vi "Main.vi"() -> ()   [LabVIEW 2015]
doc: "The boiler controller allows a user to start and shut down a boiler.\n\nUse the Reset, Start, and Light Pilot controls to sequentially start the boiler. \nUse the Fuel Control Valve to change the flow of fuel into the boiler. \nUse the Stop Boiler button to shut down the boiler. \nTo shut down the system or in the event of an emergency, use the Emergency Stop button to close the application completely."
uses:
  controls/MHL Data.ctl
  controls/MHL UI Data.ctl
  controls/MHL Status.ctl
  controls/MHL References.ctl
  controls/MHL Configuration.ctl
  support/Boiler System Globals.vi
  support/Message Queue/Message Queue.lvlib
  support/User Event - Stop/User Event - Stop.lvlib
  Boiler/Boiler.lvlib
panel:
  in  "Fuel Control Valve":u32(slide) scale=10.0..75.0
  in  "Stop Boiler":bool
  in  "Light Pilot":bool
  out "Forced Draft Fan":bool
  out "Pilot":bool
  out "Pilot Gas Valve":bool
  out "Primary Fan":bool
  out "Status":string
  in  "Start":bool
  in  "Reset":bool
  in  "Emergency Stop":bool
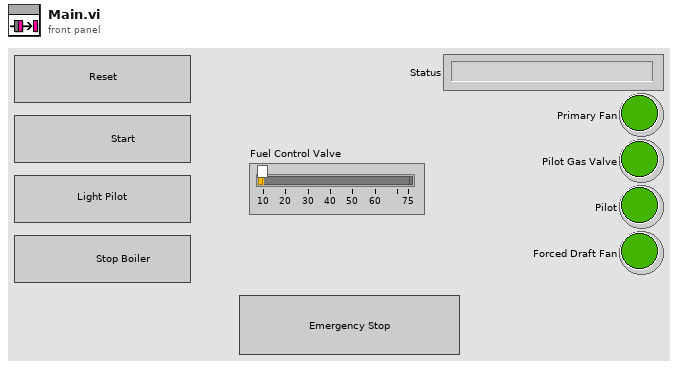
[diagram p1: front panel]
types:
  T1 = typedef "MHL Data.ctl" = cluster{"MHL User Interface Data":T2, "MHL References":T4, "MHL Configuration":T5}
  T2 = typedef "MHL UI Data.ctl" = cluster{"Status":string, "Fuel Control Valve":u32, "Primary Fan":bool, "Pilot Gas Valve":bool, "Pilot":bool, "Forced Draft Fan":bool, "MHL Status":T3}
  T3 = typedef "MHL Status.ctl" = enum16{"Lockout", "Ready", "Pre-Purge", "Pre-Purge Complete", "Pilot On", "Boiler Running", "Shutdown", "Purge"}
  T4 = typedef "MHL References.ctl" = cluster{"Reset Ref":refnum<vi>, "Start Ref":refnum<vi>, "Light Pilot Ref":refnum<vi>, "Stop Boiler Ref":refnum<vi>, "Fuel Control Valve Ref":refnum<vi>}
  T5 = typedef "MHL Configuration.ctl" = cluster{"Fuel Control Valve Maximum":dbl, "Fuel Control Valve Minimum":dbl}
  T6 = typedef "Notifiers.ctl" = cluster{"Handshake":refnum<notifier>, "Flame Level":refnum<notifier>, "Controller Exit":refnum<notifier>, "Boiler Exit":refnum<notifier>}
  T7 = typedef "Message Queue.lvlib/All Message Queues.ctl" = cluster{"MHL":refnum<queue>, "Boiler Controller":refnum<queue>, "Boiler":refnum<queue>}
  T8 = enum32{"invalid app kind", "Development System", "Run Time System", "Student Edition", "Embedded LabVIEW", "Evaluation", "Custom"}
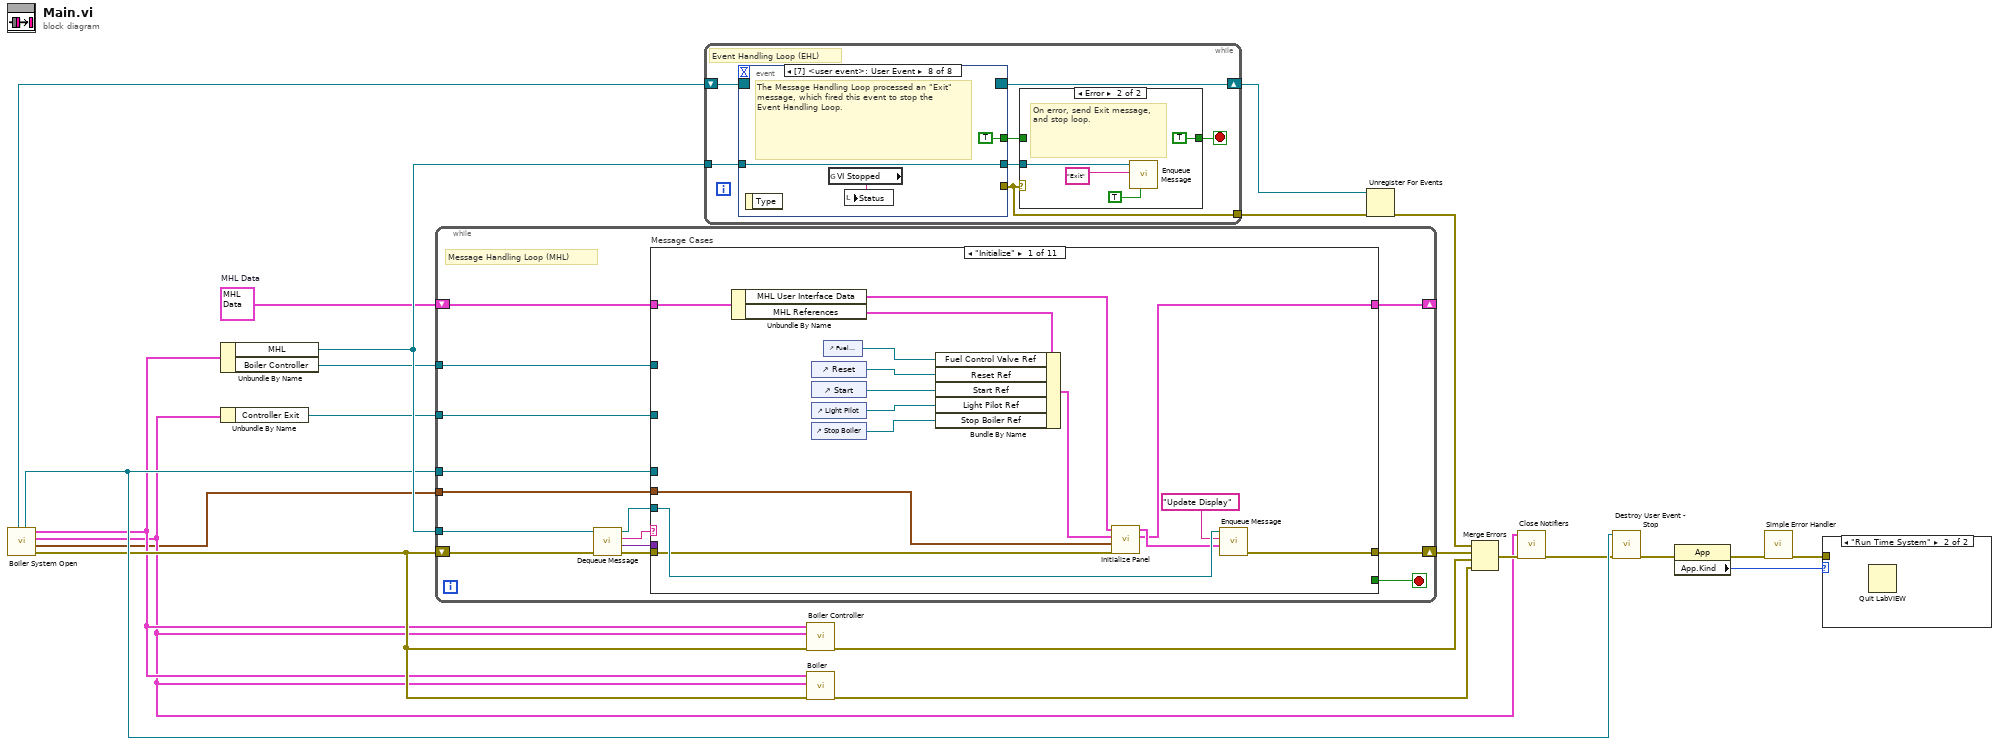
[diagram p0: block diagram]
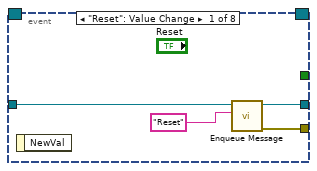
[diagram p4: hidden frame]
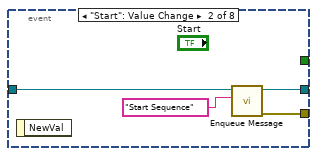
[diagram p5: hidden frame]
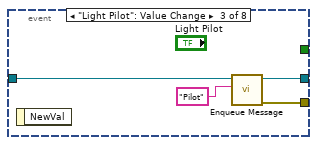
[diagram p6: hidden frame]
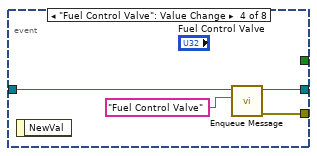
[diagram p7: hidden frame]
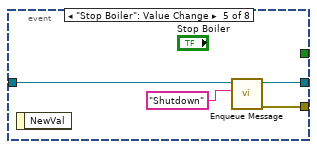
[diagram p8: hidden frame]
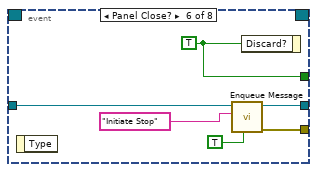
[diagram p9: hidden frame]
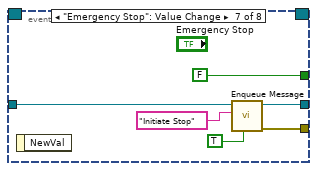
[diagram p10: hidden frame]
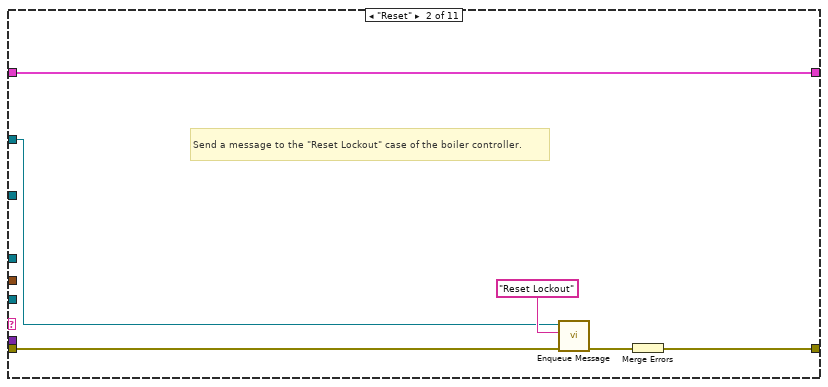
[diagram p11: hidden frame]
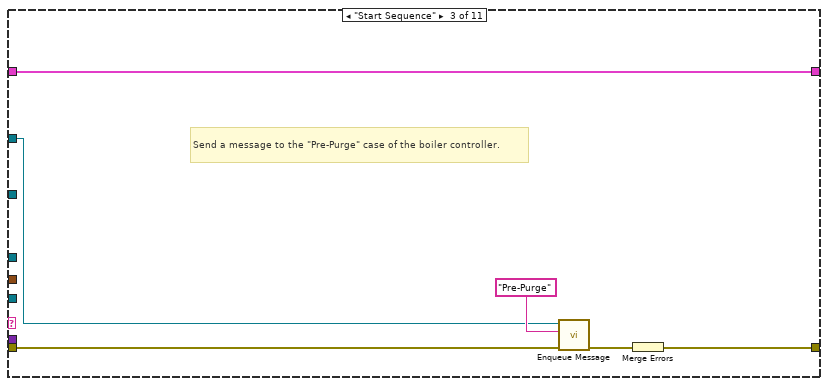
[diagram p12: hidden frame]
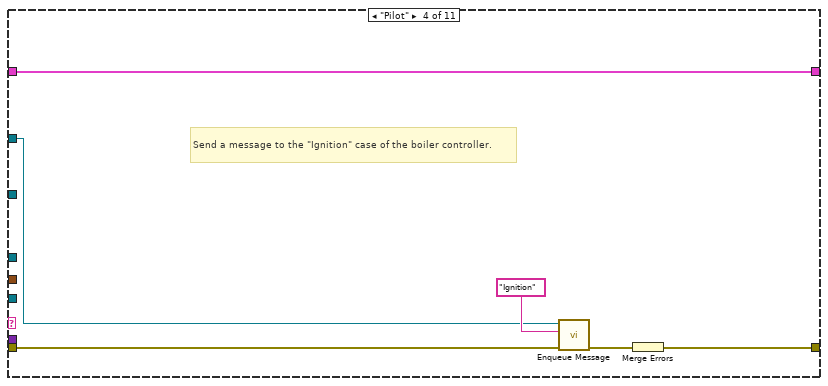
[diagram p13: hidden frame]
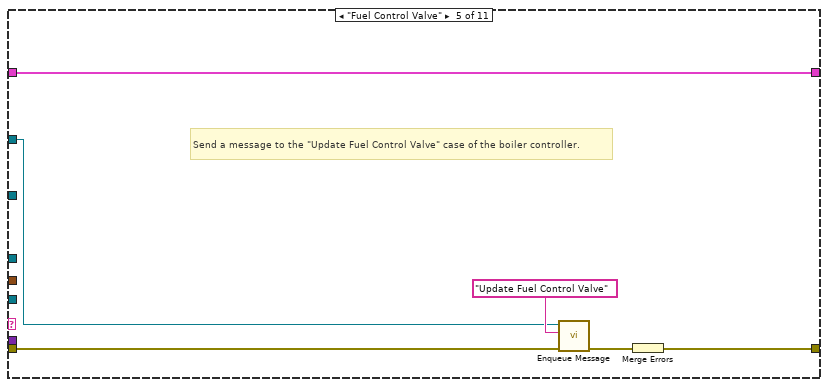
[diagram p14: hidden frame]
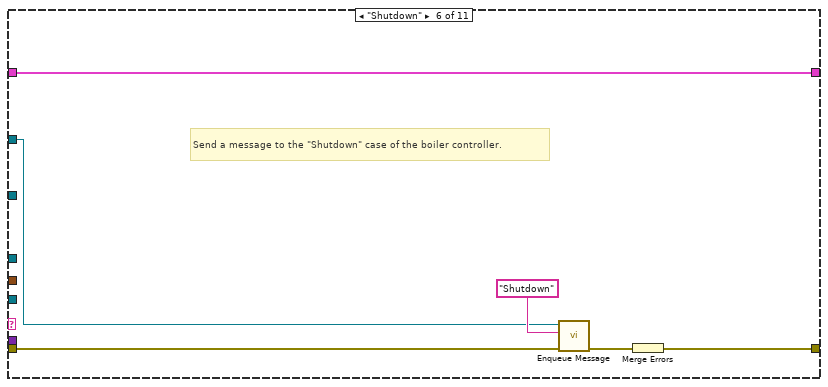
[diagram p15: hidden frame]
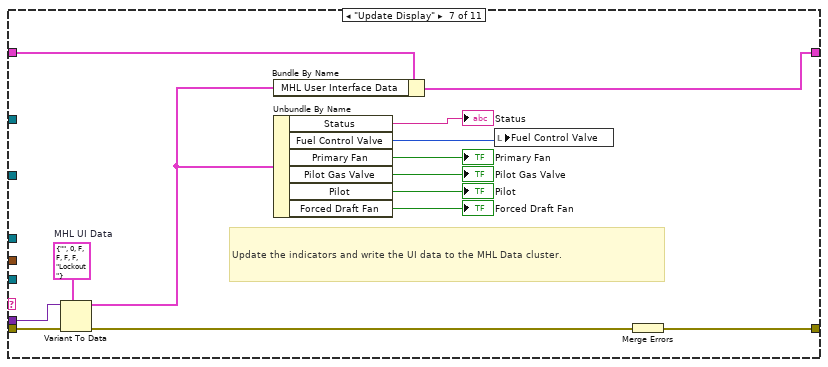
[diagram p16: hidden frame]
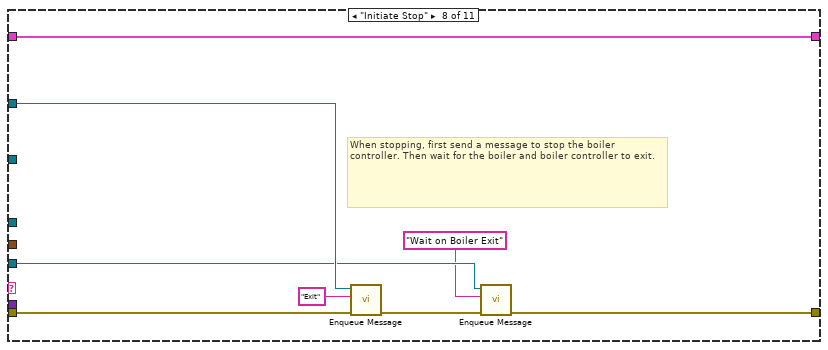
[diagram p17: hidden frame]
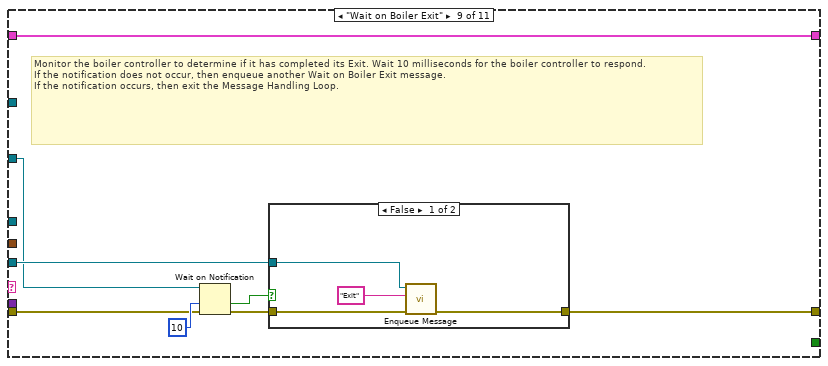
[diagram p18: hidden frame]
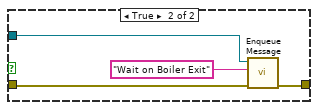
[diagram p19: hidden frame]
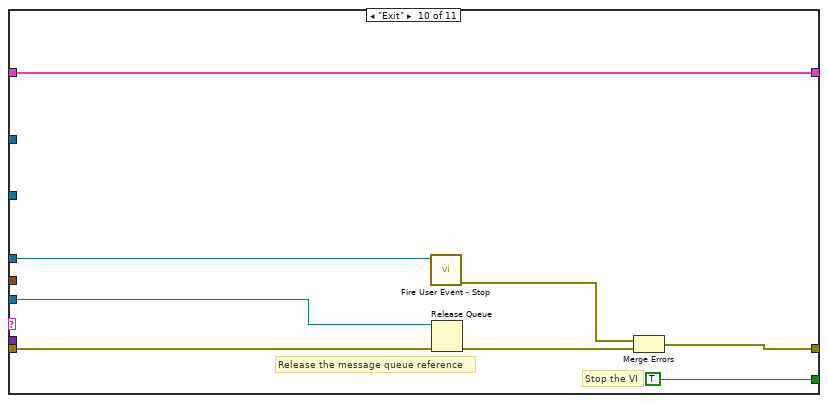
[diagram p20: hidden frame]
diagram:
  w16 = T1 {"MHL User Interface Data"={"Status"="", "Fuel Control Valve"=0, "Primary Fan"=FALSE, "Pilot Gas Valve"=FALSE, "Pilot"=FALSE, "Forced Draft Fan"=FALSE, "MHL Status"=enum."Lockout"}, "MHL References"={"Reset Ref"=refnum, "Start Ref"=refnum, "Light Pilot Ref"=refnum, "Stop Boiler Ref"=refnum, "Fuel Control Valve Ref"=refnum}, "MHL Configuration"={"Fuel Control Valve Maximum"=0.0, "Fuel Control Valve Minimum"=0.0}}  # MHL Data
  n1 = call "Boiler System Open.vi"() -> ("error out"=w7:errorcluster, "MHL Configuration"=w1:T5, "Notifiers"=w2:T6, "Message Queues"=w6:T7, "User Event - Stop"=w9:refnum<user-event>, "Stop Event Registration Refnum"=w10:refnum<event-registration>)  [unwired: 6 in]
  n2 = Unbundle By Name(w6) -> ("MHL"=w21:refnum<queue>, "Boiler Controller"=w14:refnum<queue>)
  n3 = Unbundle By Name(w2) -> ("Controller Exit"=w8:refnum<notifier>)
  n4 = while {
    tunnel: w21 -> [w26]
    shift-right: [w35] -> _
    shift-left: w16 -> [w36]
    tunnel: w9 -> [w32]
    shift-right: [w33] -> w22
    shift-left: w7 -> [w31]
    tunnel: w14 -> [w25]
    tunnel: w8 -> [w24]
    tunnel: w1 -> [w23]
    stop <- w34 stop-if-true
    # "Message Handling Loop (MHL)"
    n5 = call "Dequeue Message.vi"("error in (no error)"=w31, "Message Queue"=w26) -> ("error out"=w30:errorcluster, "Message Data"=w28:variant, "Message"=w29:string, "dup Message Queue"=w27:refnum<queue>)  [unwired: 6 in]
    n6 = case "Message Cases" shown="\"Initialize\"" w29 {
      selector: w29 -> [_ _ _ _ _ _ _ _ _ _ w132]
      tunnel: w27 -> [w45 _ _ _ _ _ _ w99 w106 w128 _]
      tunnel: w30 -> [w42 w56 w62 w68 w74 w80 w95 w104 w108 w121 _]
      tunnel: [w46 w57 w63 w69 w75 w81 w96 w101 w107 w124 w130] -> w33
      tunnel: w36 -> [w47 w58 w64 w70 w76 w82 w85 w103 w112 w127 w134]
      tunnel: [w37 w58 w64 w70 w76 w82 w83 w103 w112 w127 w134] -> w35
      tunnel: [_ _ _ _ _ _ _ _ _ TRUE _] -> w34
      tunnel: w28 -> [_ _ _ _ _ _ w94 _ _ _ _]
      tunnel: w32 -> [_ _ _ _ _ _ _ _ _ w123 _]
      tunnel: w25 -> [_ w53 w59 w65 w71 w77 _ w100 _ _ _]
      tunnel: w24 -> [_ _ _ _ _ _ _ _ w105 _ _]
      tunnel: w23 -> [w41 _ _ _ _ _ _ _ _ _ _]
      frame "Initialize" {
        n7 = Unbundle By Name(w47) -> ("MHL User Interface Data"=w39:T2, "MHL References"=w43:T4)
        n8 = control-ref of="Reset"() -> (w49:refnum<vi>)
        n9 = control-ref of="Start"() -> (w50:refnum<vi>)
        n10 = control-ref of="Light Pilot"() -> (w51:refnum<vi>)
        n11 = control-ref of="Stop Boiler"() -> (w52:refnum<vi>)
        n12 = control-ref of="Fuel Control Valve"() -> (w48:refnum<vi>)
        n13 = Bundle By Name(cluster=w43, "Fuel Control Valve Ref"=w48, "Reset Ref"=w49, "Start Ref"=w50, "Light Pilot Ref"=w51, "Stop Boiler Ref"=w52) -> (w40:T4)
        n14 = call "Initialize Panel.vi"("error in"=w42, "MHL Configuration"=w41, "MHL References"=w40, "MHL UI Data in"=w39) -> ("MHL Data out"=w37:T1, "MHL UI Data out"=w38:T2)  [unwired: 5 in, 1 out]
        n15 = call "Enqueue Message.vi"("Message Data"=w38, "Message"="Update Display", "Message Queue"=w45) -> ("error out"=w46:errorcluster)  [unwired: 7 in, 1 out]
      }
      frame "Reset" {
        # "Send a message to the \"Reset Lockout\" case of the boiler controller."
        n16 = call "Enqueue Message.vi"("error in (no error)"=w56, "Message"="Reset Lockout", "Message Queue"=w53) -> ("error out"=w55:errorcluster)  [unwired: 7 in, 1 out]
        n17 = Merge Errors(w55) -> (w57:errorcluster)
      }
      frame "Start Sequence" {
        # "Send a message to the \"Pre-Purge\" case of the boiler controller."
        n18 = call "Enqueue Message.vi"("error in (no error)"=w62, "Message"="Pre-Purge", "Message Queue"=w59) -> ("error out"=w61:errorcluster)  [unwired: 7 in, 1 out]
        n19 = Merge Errors(w61) -> (w63:errorcluster)
      }
      frame "Pilot" {
        # "Send a message to the \"Ignition\" case of the boiler controller."
        n20 = call "Enqueue Message.vi"("error in (no error)"=w68, "Message"="Ignition", "Message Queue"=w65) -> ("error out"=w67:errorcluster)  [unwired: 7 in, 1 out]
        n21 = Merge Errors(w67) -> (w69:errorcluster)
      }
      frame "Fuel Control Valve" {
        # "Send a message to the \"Update Fuel Control Valve\" case of the boiler controller."
        n22 = call "Enqueue Message.vi"("error in (no error)"=w74, "Message"="Update Fuel Control Valve", "Message Queue"=w71) -> ("error out"=w73:errorcluster)  [unwired: 7 in, 1 out]
        n23 = Merge Errors(w73) -> (w75:errorcluster)
      }
      frame "Shutdown" {
        # "Send a message to the \"Shutdown\" case of the boiler controller."
        n24 = call "Enqueue Message.vi"("error in (no error)"=w80, "Message"="Shutdown", "Message Queue"=w77) -> ("error out"=w79:errorcluster)  [unwired: 7 in, 1 out]
        n25 = Merge Errors(w79) -> (w81:errorcluster)
      }
      frame "Update Display" {
        w92 = T2 {"Status"="", "Fuel Control Valve"=0, "Primary Fan"=FALSE, "Pilot Gas Valve"=FALSE, "Pilot"=FALSE, "Forced Draft Fan"=FALSE, "MHL Status"=enum."Lockout"}  # MHL UI Data
        # "Update the indicators and write the UI data to the MHL Data cluster."
        n26 = Variant To Data(error in=w95, type=w92, Variant=w94) -> (data=w84:T2, error out=w93:errorcluster)
        n27 = Bundle By Name(cluster=w85, "MHL User Interface Data"=w84) -> (w83:T1)
        n28 = Unbundle By Name(w84) -> ("Status"=→"Status":string, "Fuel Control Valve"=w90:u32, "Primary Fan"=→"Primary Fan":bool, "Pilot Gas Valve"=→"Pilot Gas Valve":bool, "Pilot"=→"Pilot":bool, "Forced Draft Fan"=→"Forced Draft Fan":bool)
        n29 = local write "Fuel Control Valve"(w90) -> ()
        n30 = Merge Errors(w93) -> (w96:errorcluster)
      }
      frame "Initiate Stop" {
        # "When stopping, first send a message to stop the boiler controller. Then wait for the boiler and boiler controller to exit."
        n31 = call "Enqueue Message.vi"("error in (no error)"=w104, "Message"="Exit", "Message Queue"=w100) -> ("error out"=w102:errorcluster)  [unwired: 7 in, 1 out]
        n32 = call "Enqueue Message.vi"("error in (no error)"=w102, "Message"="Wait on Boiler Exit", "Message Queue"=w99) -> ("error out"=w101:errorcluster)  [unwired: 7 in, 1 out]
      }
      frame "Wait on Boiler Exit" {
        # "Monitor the boiler controller to determine if it has completed its Exit. Wait 10 milliseconds for the boiler controller to respond. \nIf the notification does not occur, then enqueue another Wait on Boiler Exit message.\nIf the notification occurs, then exit the Message Handling Loop."
        n33 = Wait on Notification(notifier=w105, timeout in ms (-1)=10, error in (no error)=w108) -> (timed out?=w110:bool, error out=w109:errorcluster)  [unwired: 1 in, 2 out]
        n34 = case shown="False" w110 {
          tunnel: w109 -> [w116 w120]
          tunnel: w106 -> [w115 w118]
          tunnel: [w113 w119] -> w107
          frame False {
            n35 = call "Enqueue Message.vi"("error in (no error)"=w116, "Message"="Exit", "Message Queue"=w115) -> ("error out"=w113:errorcluster)  [unwired: 7 in, 1 out]
          }
          frame True {
            n36 = call "Enqueue Message.vi"("error in (no error)"=w120, "Message"="Wait on Boiler Exit", "Message Queue"=w118) -> ("error out"=w119:errorcluster)  [unwired: 7 in, 1 out]
          }
        }
      }
      frame "Exit" {
        # "Stop the VI"
        # "Release the message queue reference"
        n37 = call "Fire User Event - Stop.vi"("User Event - Stop"=w123) -> ("error out"=w122:errorcluster)  [unwired: 10 in]
        n38 = Release Queue(queue=w128, error in (no error)=w121) -> (error out=w125:errorcluster)  [unwired: 1 in, 2 out]
        n39 = Merge Errors(w122, w125) -> (w124:errorcluster)
      }
      frame Default {
        # "'Default' case only runs if there is a message that isn't defined in any of the other cases.  Output a programming error."
        n40 = Format Into String(format string="The invalid message string \"%s\" was received in the Message Handling Loop." ("Unknown Message Error Text"), w132) -> (resulting string=w129:string)  [unwired: 2 in, 1 out]
        n41 = call <vilib>:"Error Cluster From Error Code.vi"("error message (\"\")"=w129, "error code (0)"=1) -> ("error out"=w130:errorcluster)  [unwired: 7 in]
      }
    }
  }
  n42 = while {
    tunnel: w21 -> [w141]
    tunnel: [w137] -> w18
    shift-right: [w135] -> w17
    shift-left: w10 -> [w136]
    stop <- w139 stop-if-true
    # "Event Handling Loop (EHL)"
    n43 = event shown="[7] <user event>: User Event" {
      selector: w136 -> [_ _ _ _ _ _ _ _]
      dyn-events: [_ _ _ _ _ _ _ _] -> w135
      timeout: _ -> [_ _ _ _ _ _ _ _]
      tunnel: [_ _ _ _ _ w172 FALSE ("Discard?") TRUE ("Discard?")] -> w140
      tunnel: w141 -> [w150 w154 w158 w162 w166 w171 w178 w181]
      tunnel: [w149 w152 w156 w160 w164 w170 w177 _] -> w137
      tunnel: [w148 w153 w157 w161 w165 w169 w175 w181] -> w138
      event "Reset": Value Change {
        n44 = event-data() -> ()  [unwired: 1 in, 1 out]
        n45 = call "Enqueue Message.vi"("Message"="Reset", "Message Queue"=w150) -> ("error out"=w149:errorcluster, "dup Message Queue"=w148:refnum<queue>)  [unwired: 8 in]
      }
      event "Start": Value Change {
        n46 = event-data() -> ()  [unwired: 1 in, 1 out]
        n47 = call "Enqueue Message.vi"("Message"="Start Sequence", "Message Queue"=w154) -> ("error out"=w152:errorcluster, "dup Message Queue"=w153:refnum<queue>)  [unwired: 8 in]
      }
      event "Light Pilot": Value Change {
        n48 = event-data() -> ()  [unwired: 1 in, 1 out]
        n49 = call "Enqueue Message.vi"("Message"="Pilot", "Message Queue"=w158) -> ("error out"=w156:errorcluster, "dup Message Queue"=w157:refnum<queue>)  [unwired: 8 in]
      }
      event "Fuel Control Valve": Value Change {
        n50 = event-data() -> ()  [unwired: 1 in, 1 out]
        n51 = call "Enqueue Message.vi"("Message"="Fuel Control Valve", "Message Queue"=w162) -> ("error out"=w160:errorcluster, "dup Message Queue"=w161:refnum<queue>)  [unwired: 8 in]
      }
      event "Stop Boiler": Value Change {
        n52 = event-data() -> ()  [unwired: 1 in, 1 out]
        n53 = call "Enqueue Message.vi"("Message"="Shutdown", "Message Queue"=w166) -> ("error out"=w164:errorcluster, "dup Message Queue"=w165:refnum<queue>)  [unwired: 8 in]
      }
      event Panel Close? {
        w172 = TRUE ("Discard?")
        n54 = event-data() -> ()  [unwired: 1 in, 1 out]
        n55 = call "Enqueue Message.vi"("Priority Message? (F)"=TRUE, "Message"="Initiate Stop", "Message Queue"=w171) -> ("error out"=w170:errorcluster, "dup Message Queue"=w169:refnum<queue>)  [unwired: 7 in]
        n56 = event-data("Discard?"=w172) -> ()  [unwired: 1 in, 1 out]
      }
      event "Emergency Stop": Value Change {
        n57 = event-data() -> ()  [unwired: 1 in, 1 out]
        n58 = call "Enqueue Message.vi"("Priority Message? (F)"=TRUE, "Message"="Initiate Stop", "Message Queue"=w178) -> ("error out"=w177:errorcluster, "dup Message Queue"=w175:refnum<queue>)  [unwired: 7 in]
      }
      event User Event {
        # "The Message Handling Loop processed an \"Exit\" message, which fired this event to stop the Event Handling Loop."
        n59 = event-data() -> ()  [unwired: 1 in, 1 out]
        n60 = global read "Boiler System Globals.vi" "VI Stopped"() -> (w179:string)
        n61 = local write "Status"(w179) -> ()
      }
    }
    n62 = case shown="Error" w137 {
      tunnel: [w142 TRUE ("Discard?")] -> w139
      tunnel: w140 -> [w142 _]
      tunnel: w138 -> [_ w145]
      frame No Error {
      }
      frame Error {
        # "On error, send Exit message, and stop loop."
        n63 = call "Enqueue Message.vi"("Priority Message? (F)"=TRUE, "Message"="Exit", "Message Queue"=w145) -> ()  [unwired: 7 in, 2 out]
      }
    }
  }
  n64 = call "Boiler Controller.vi"("error in"=w7, "Notifiers"=w2, "Message Queues"=w6) -> ("error out"=w15:errorcluster)  [unwired: 8 in]
  n65 = call "Boiler.vi"("error in"=w7, "Notifiers"=w2, "Message Queues"=w6) -> ("error out"=w5:errorcluster)  [unwired: 8 in]
  n66 = Unregister For Events(event registration refnum=w17, error in=w18) -> (error out=w19:errorcluster)
  n67 = Merge Errors(w19, w22, w15, w5) -> (w4:errorcluster)
  n68 = call "Close Notifiers.vi"("error in"=w4, "Notifiers"=w2) -> ("error out"=w3:errorcluster)  [unwired: 9 in]
  n69 = call "Destroy User Event - Stop.vi"("error in (no error)"=w3, "User Event - Stop"=w9) -> ("error out"=w20:errorcluster)  [unwired: 9 in]
  n70 = property class="App"(error in=w20) -> (error out=w13:errorcluster, "App.Kind"=w12:T8)  [unwired: 1 in, 1 out]
  n71 = call <vilib>:"Simple Error Handler.vi"("error in (no error)"=w13) -> ("error out"=w11:errorcluster)  [unwired: 4 in, 4 out]
  n72 = case shown="\"Run Time System\"" w12 {
    tunnel: w11 -> [_ _]
    frame Default {
    }
    frame "Run Time System" {
      n73 = Quit LabVIEW() -> ()  [unwired: 1 in]
    }
  }
